vi "G#RealTimeTemplate_Kernel.vi"(0 "reference in":refnum<class "G#RealTimeTemplate.lvclass">, 1 "New? (F=Dispose)":bool, 5 "error in (no error)":errorcluster) -> (14 "reference out":refnum<class "G#RealTimeTemplate.lvclass">, 19 "error out":errorcluster)   [LabVIEW 2020, in "G#RealTimeTemplate.lvclass"]
doc: "Returns a reference and if wanted the actual data values of the attributes. This method is used by the subclasses to access parent attributes."
uses:
  <vilib>/addons/_AddQ/G#Templates/G#RealTimeTemplate/G#RealTimeTemplate.lvclass
  <vilib>/addons/_AddQ/G#Templates/G#RealTimeTemplate/utils/ObjectAttributesRef.ctl
  <vilib>/addons/_AddQ/G#Templates/G#RealTimeTemplate/protected/ObjectAttributes.ctl
  <vilib>/addons/_AddQ/G#Templates/G#RealTimeTemplate/G#RealTimeTemplate.lvclass/G#RealTimeTemplate.ctl
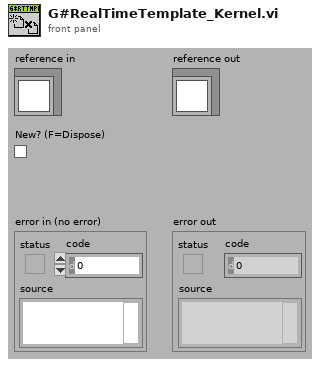
[diagram p1: front panel]
types:
  T1 = typedef "G#RealTimeTemplate.lvclass/ObjectAttributesRef.ctl" = refnum<data-value>
  T2 = typedef "G#RealTimeTemplate.lvclass/ObjectAttributes.ctl" = cluster{"MyAttribute":dbl}
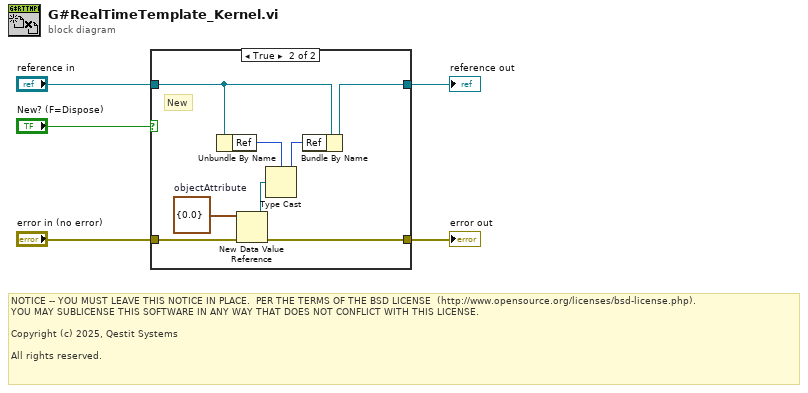
[diagram p0: block diagram]
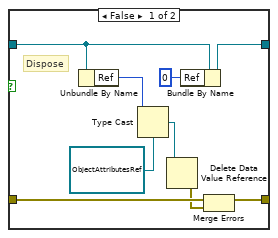
[diagram p2: hidden frame]
diagram:
  # "NOTICE -- YOU MUST LEAVE THIS NOTICE IN PLACE.  PER THE TERMS OF THE BSD LICENSE  (http://www.opensource.org/licenses/bsd-license.php).\nYOU MAY SUBLICENSE THIS SOFTWARE IN ANY WAY THAT DOES NOT CONFLICT WITH THIS LICENSE.\n\nCopyright (c) 2025, Qestit Systems\n\nAll rights reserved."
  n1 = case shown="True" "New? (F=Dispose)" {
    tunnel: "error in (no error)" -> [w14 w17]
    tunnel: [w13 w16] -> w4
    tunnel: "reference in" -> [w12 w18]
    tunnel: [w11 w15] -> w2
    frame False {
      # "Dispose"
      n2 = Unbundle By Name(w12) -> ("Ref"=w10:u32)
      n3 = Type Cast(type=T1 refnum ("attributes ref"), x=w10) -> (*(type *) &x=w8:T1)
      n4 = Delete Data Value Reference(data value reference=w8) -> (error out=w7:errorcluster)  [unwired: 1 in, 1 out]
      n5 = Bundle By Name(cluster=w12, "Ref"=u32 0) -> (w11:refnum<class "G#RealTimeTemplate.lvclass">)
      n6 = Merge Errors(w14, w7) -> (w13:errorcluster)
    }
    frame True {
      w22 = T2 {"MyAttribute"=0.0}  # objectAttribute
      # "New"
      n7 = Unbundle By Name(w18) -> ("Ref"=w20:u32)
      n8 = New Data Value Reference(data value=w22, error in=w17) -> (data value reference=w19:refnum<data-value>, error out=w16:errorcluster)
      n9 = Type Cast(type=w20, x=w19) -> (*(type *) &x=w21:u32)
      n10 = Bundle By Name(cluster=w18, "Ref"=w21) -> (w15:refnum<class "G#RealTimeTemplate.lvclass">)
    }
  }
  "error out" <- w4
  "reference out" <- w2
